vi "Write 1Chan NSamp 1D SGL.vi"(8 "error in (no error)":errorcluster, 10 "data":sgl[](array[numeric]), 11 "Analog Output in":refnum<class "Analog output.lvclass">) -> (0 "error out":errorcluster, 3 "Analog Output out":refnum<class "Analog output.lvclass">)   [LabVIEW 2009, in "MicroDAQ.lvlib" / "Analog output.lvclass"]
doc: "Writes buffor of floating-points samples to channel."
uses:
  <instrlib>/MicroDAQ/Channel/Analog Output/Analog output.lvclass
  <instrlib>/MicroDAQ/Channel/Analog Output/Analog output.lvclass/Analog output.ctl
  <instrlib>/MicroDAQ/Channel/Channel.lvclass
  <instrlib>/MicroDAQ/Mlink library wraper/mlink.lvlib
  <instrlib>/MicroDAQ/MicroDAQ.lvlib
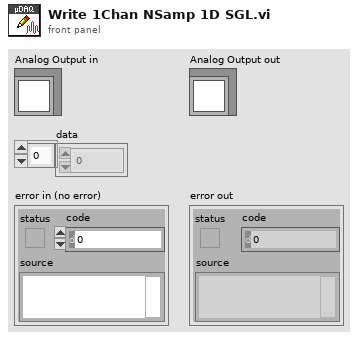
[diagram p1: front panel]
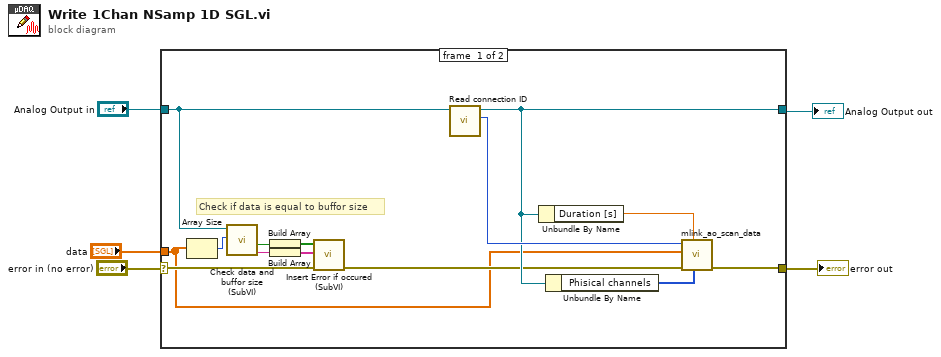
[diagram p0: block diagram]
diagram:
  n1 = case shown="No Error" "error in (no error)" {
    selector: "error in (no error)" -> [w9 w21]
    tunnel: [w19 w21] -> w4
    tunnel: [w16 w20] -> w1
    tunnel: "Analog Output in" -> [w14 w20]
    tunnel: "data" -> [w6 _]
    frame #0 {
      # "Check if data is equal to buffor size"
      n2 = Array Size(array=w6) -> (size(s)=w7:i32)
      n3 = call <instrlib>:"Check data and buffor size (SubVI).vi"("data size"=w7, "Analog output in"=w14) -> ("Error message"=w12:string, "Error?"=w13:bool)  [unwired: 8 in]
      n4 = Build Array(w13) -> (w11:bool[])
      n5 = Build Array(w12) -> (w10:string[])
      n6 = call <instrlib>:"Insert Error if occured (SubVI).vi"("error in (no error)"=w9, "Error messages"=w10, "Error conditionals"=w11) -> ("error out"=w8:errorcluster)  [unwired: 8 in]
      n7 = call <instrlib>:"Read connection ID.vi"("Task in"=w14) -> ("connection ID"=w18:i32, "Task out"=w16:refnum<class "Analog output.lvclass">)  [unwired: 9 in]
      n8 = Unbundle By Name(w16) -> ("Duration [s]"=w15:dbl)
      n9 = Unbundle By Name(w16) -> ("Phisical channels"=w17:u8[])
      n10 = call <instrlib>:"mlink_ao_scan_data.vi"("channels"=w17, "opt"=w15, "error in (no error)"=w8, "data"=w6, "connection ID"=w18) -> ("error out"=w19:errorcluster)  [unwired: 5 in, 1 out]
    }
    frame #1 {
    }
  }
  "error out" <- w4
  "Analog Output out" <- w1
